vi "Calc_Turret.vi"(10 "Turret Command Inputs":T2, 11 "Turret Sensor Inputs":T1) -> (3 "Turret Outputs":T3)   [LabVIEW 2012]
uses:
  Outputs_Turret.ctl
  Inputs_Commands_Turret.ctl
  Inputs_Sensors_Turret.ctl
panel:
  in  "Physical Deadband":dbl=0.1
  in  "Zero Tolerance":dbl=0.01
  out "error out":errorcluster
  in  "D":dbl
  in  "I":dbl
  in  "P":dbl
  in  "Set PID":bool
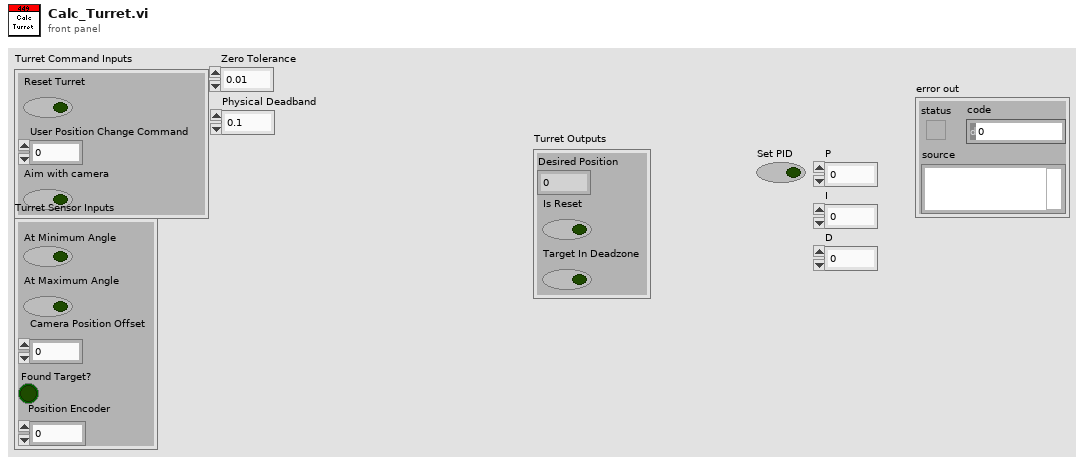
[diagram p1: front panel]
types:
  T1 = typedef "Inputs_Sensors_Turret.ctl" = cluster{"At Minimum Angle":bool, "At Maximum Angle":bool, "Camera Position Offset":dbl, "Found Target?":bool, "Position Encoder":dbl}
  T2 = typedef "Inputs_Commands_Turret.ctl" = cluster{"Reset Turret":bool, "User Position Change Command":dbl, "Aim with camera":bool}
  T3 = typedef "Outputs_Turret.ctl" = cluster{"Desired Position":dbl, "Is Reset":bool, "Target In Deadzone":bool}
  T4 = typedef "WPI_MotorControlDeviceRef.ctl" = cluster{"DeviceStatus":errorcluster, "Type":enum16{"PWM", "CAN"}, "PWM":cluster{"Digital Module":T5, "PWM Channel":T6, "DeadBand":T7}, "CAN":cluster{"Device Number":u8, "Control Mode":T8, "Semaphore":T9, "Max Vout":dbl}, "Invert":bool, "TransformRef":T10, "InvTransformRef":T10}
  T5 = typedef "FPGA_TypedefDigitalModule.ctl" = enum16{"Digital Module 1", "Digital Module 2"}
  T6 = typedef "FPGA_DIOPWMChannel.ctl" = enum8{"PWM 1", "PWM 2", "PWM 3", "PWM 4", "PWM 5", "PWM 6", "PWM 7", "PWM 8", "PWM 9", "PWM 10", "Invalid"}
  T7 = typedef "WPI_PWMDeadband.ctl" = cluster{"Name":string, "maxPositivePwm":i32, "minPositivePwm":i32, "centerPwm":i32, "maxNegativePwm":i32, "minNegativePwm":i32, "angularRange":u16}
  T8 = typedef "WPI_CANJaguar_ControlMode.ctl" = enum8{"Percent VBus", "Current", "Speed", "Position", "Voltage"}
  T9 = typedef "Semaphore RefNum" = refnum<k1>
  T10 = typedef "WPI_PWMTransform_ConPane.ctl" = refnum<vi>
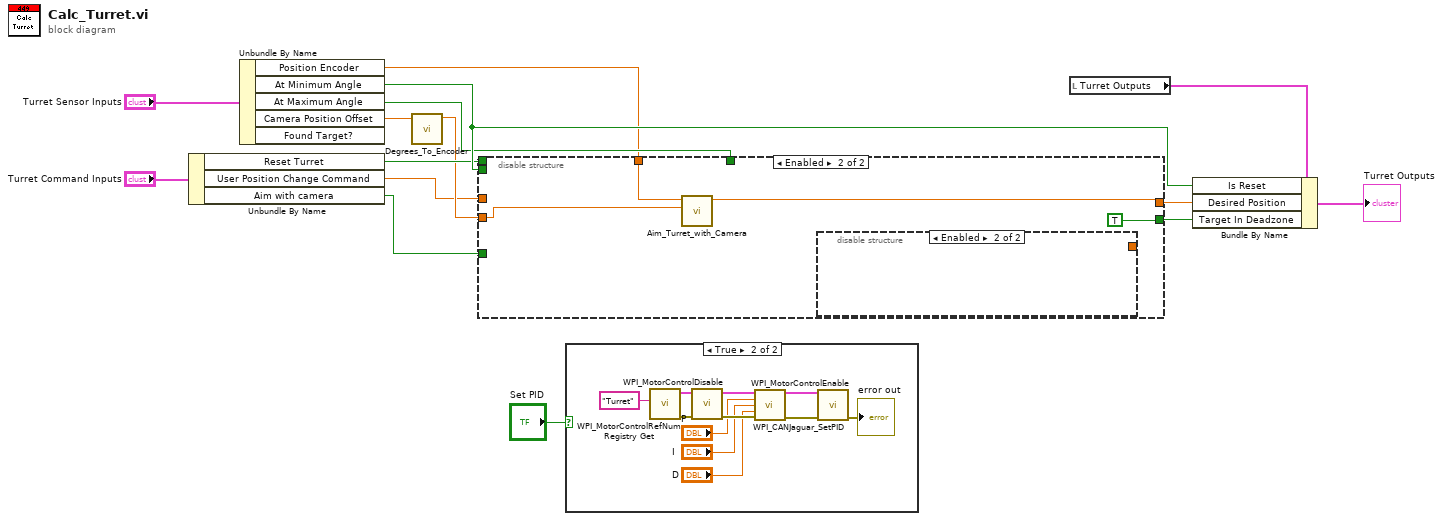
[diagram p0: block diagram]
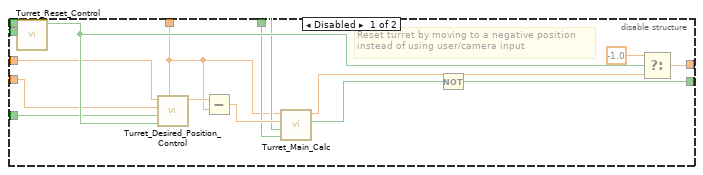
[diagram p2: hidden frame]
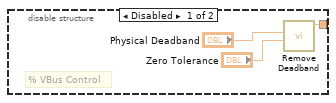
[diagram p3: hidden frame]
diagram:
  n1 = Unbundle By Name("Turret Command Inputs") -> ("Reset Turret"=w6:bool, "User Position Change Command"=w2:dbl, "Aim with camera"=w5:bool)
  n2 = Unbundle By Name("Turret Sensor Inputs") -> ("Position Encoder"=w1:dbl, "At Minimum Angle"=w8:bool, "At Maximum Angle"=w7:bool, "Camera Position Offset"=w4:dbl)  [unwired: 1 out]
  n3 = call "Degrees_To_Encoder.vi"("Degree Value"=w4) -> ("Encoder Value"=w3:dbl)  [unwired: 10 in]
  n4 = disable-structure shown="Enabled" {
    disable-tunnel: [w16 TRUE] -> w13
    disable-tunnel: [w24 w31] -> w12
    disable-tunnel: w8 -> [w23 _]
    disable-tunnel: w7 -> [w22 _]
    disable-tunnel: w6 -> [w21 _]
    disable-tunnel: w5 -> [w20 _]
    disable-tunnel: w3 -> [w18 w32]
    disable-tunnel: w2 -> [w19 _]
    disable-tunnel: w1 -> [w17 w33]
    frame Disabled {
      # "Reset turret by moving to a negative position\ninstead of using user/camera input"
      n5 = call "Turret_Reset_Control.vi"("Turret Is Reset"=w23, "Reset Turret Command"=w21) -> ("Reset Turret Output"=w26:bool)  [unwired: 9 in]
      n6 = call "Turret_Desired_Position_Control.vi"("Current Position"=w17, "Reset Turret?"=w26, "Aim with Camera?"=w20, "Camera Desired Position Change"=w18, "User Position Change Command"=w19) -> ("Desired Position"=w30:dbl)  [unwired: 6 in]
      n7 = Subtract(x=w30, y=w17) -> (x-y=w29:dbl)
      n8 = call "Turret_Main_Calc.vi"("At Maximum Angle"=w22, "At Minimum Angle"=w23, "Desired Horizontal Offset"=w29, "Current Horizontal Position"=w17) -> ("Target In Deadzone"=w25:bool, "Output Turret Position"=w27:dbl)  [unwired: 6 in]
      n9 = Not(x=w25) -> (.not. x?=w16:bool)
      n10 = Select(t=-1.0, s=w26, f=w27) -> (s? t:f=w24:dbl)
    }
    frame Enabled {
      n11 = call "Aim_Turret_with_Camera.vi"("Angle Change"=w32, "Current Encoder Pos"=w33) -> ("New Encoder Pos"=w31:dbl)  [unwired: 9 in]
      n12 = disable-structure shown="Enabled" {
        disable-tunnel: [w37 _] -> _
        frame Disabled {
          # "% VBus Control"
          n13 = call "Remove Deadband.vi"("Zero Tolerance"="Zero Tolerance", "Physical Deadband"="Physical Deadband") -> ("Output without deadband"=w37:dbl)  [unwired: 9 in]
        }
        frame Enabled {
        }
      }
    }
  }
  n14 = case shown="True" "Set PID" {
    frame False {
    }
    frame True {
      n15 = call <vilib>:"WPI_MotorControlRefNum Registry Get.vi"("refnum name"="Turret") -> ("error out"=w47:errorcluster, "MotorControlDevRef"=w46:T4)  [unwired: 9 in]
      n16 = call <vilib>:"WPI_MotorControlDisable.vi"("error in (no error)"=w47, "MotorControlDevRef"=w46) -> ("error out"=w44:errorcluster, "MotorControlDevRef"=w45:T4)  [unwired: 8 in]
      n17 = call <vilib>:"WPI_CANJaguar_SetPID.vi"("CAN Jaguar Ref"=w45, "P"="P", "I"="I", "D"="D", "error in (no error)"=w44) -> ("CAN Jaguar Ref Out"=w39:T4, "error out"=w40:errorcluster)  [unwired: 9 in]
      n18 = call <vilib>:"WPI_MotorControlEnable.vi"("error in (no error)"=w40, "CAN Jaguar Ref"=w39) -> ("error out"=→"error out":errorcluster)  [unwired: 8 in, 1 out]
    }
  }
  n19 = local read "Turret Outputs"() -> (w15:T3)
  n20 = Bundle By Name(cluster=w15, "Is Reset"=w8, "Desired Position"=w12, "Target In Deadzone"=w13) -> (→"Turret Outputs":T3)
